vi "Save To Clip Board.vi"(11 "palette":string) -> (2 "function return":u32, 3 "palette out":string)   [LabVIEW 2018, in "AndorSDK.lvlib"]
doc: "EXPNETTYPE unsigned int WINAPI SaveToClipBoard(char * palette);"
uses:
  AndorSDK.lvlib
  ATMCD32D.dll
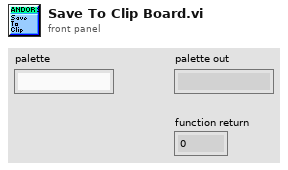
[diagram p1: front panel]
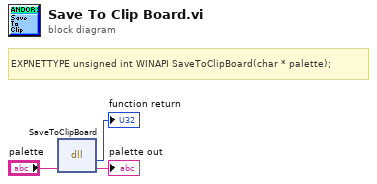
[diagram p0: block diagram]
diagram:
  # "EXPNETTYPE unsigned int WINAPI SaveToClipBoard(char * palette);"
  n1 = dll-call lib="PTH2babs E\nPersönliches02 - Arbeit03-HiwijobsLabviewCodelibANDOR\tAndor SDK\nATMCD32D.*" fn="SaveToClipBoard"("palette"="palette") -> (→"function return":u32, "palette"=→"palette out":string)  [unwired: 3 in, 2 out]
